vi "Simple Solenoid.vi"() -> ()   [LabVIEW 2018]
doc: "Simple Solenoid Example\n\nThis example shows how to set the value of a Solenoid Channel.\n\nIt works with the PCM (Pneumatic Control Module) communicating with the roboRIO over CAN bus. The PCM must also be supplied with 12V DC from the PDP (Power Distribution Panel).\n\nThe Compressor, Pressure Switch, and Solenoid are all wired to the PCM \n\nThis example expects a USB cable connected from your development PC to the Type B USB Jack (next to the power input) on the roboRIO.\n\nThis example expects the Driver Station to be running."
uses:
  <vilib>/Rock Robotics/WPI/Solenoid/WPI_SolenoidSetEnum.vi
  <vilib>/Rock Robotics/WPI/Solenoid/WPI_SolenoidValue.ctl
panel:
  in  "Value to Write 2":bool
  in  "stop 2":bool
  in  "Value to Write":bool
  in  "stop":bool
  # "Set this input before running."
  # "This can be set while running."
  # "On"
  # "Off"
  # "Wiring Diagram"
  # "Pneumatic Control Module"
  # "To Solenoid"
  # "CAN"
  # "COMPRESSOR OUT"
  # "PRESSURE"
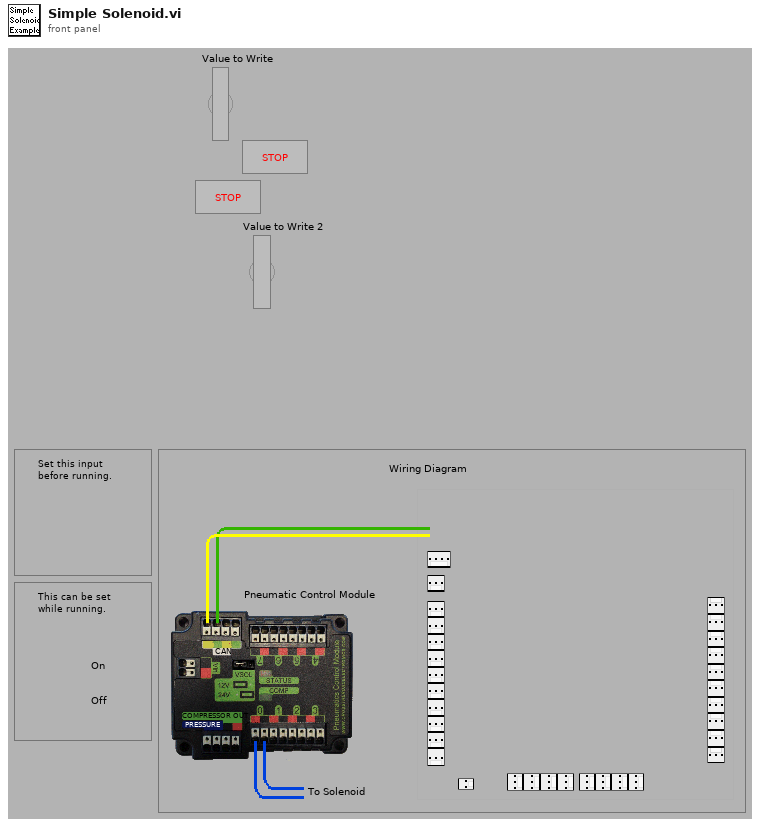
[diagram p1: front panel]
types:
  T1 = typedef "WPI_SolenoidValue.ctl" = enum16{"Off", "On", "Forward", "Reverse"}
  T2 = typedef "WPI_SolenoidDevRef.ctl" = cluster{"DevStatus":errorcluster, "Pneumatics Control Module":u8, "Forward Solenoid Channel":T3, "Reverse Solenoid Channel":T3}
  T3 = typedef "WPI_SolenoidChannel.ctl" = enum8{"Solenoid 0", "Solenoid 1", "Solenoid 2", "Solenoid 3", "Solenoid 4", "Solenoid 5", "Solenoid 6", "Solenoid 7", "Invalid"}
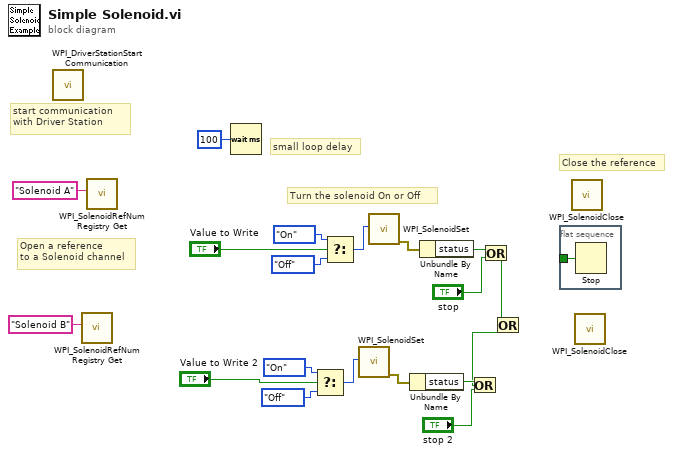
[diagram p0: block diagram]
diagram:
  # "small loop delay"
  # "Turn the solenoid On or Off"
  # "start communication with Driver Station"
  # "Close the reference"
  # "Open a reference \nto a Solenoid channel"
  n1 = call <vilib>:"WPI_DriverStationStart Communication.vi"() -> ()  [unwired: 2 in, 10 out]
  n2 = call <vilib>:"WPI_SolenoidRefNum Registry Get.vi"("refnum name"="Solenoid B") -> ("SolenoidDevRef"=w23:T2)  [unwired: 9 in, 1 out]
  n3 = call <vilib>:"WPI_SolenoidRefNum Registry Get.vi"("refnum name"="Solenoid A") -> ("SolenoidDevRef"=w26:T2)  [unwired: 9 in, 1 out]
  n4 = Wait (ms)(milliseconds to wait=u32 100) -> ()  [unwired: 1 out]
  n5 = Select(t=WPI_SolenoidValue."On" ("Value"), s="Value to Write 2", f=WPI_SolenoidValue."Off" ("Value")) -> (s? t:f=w6:T1)
  n6 = Select(t=WPI_SolenoidValue."On" ("Value"), s="Value to Write", f=WPI_SolenoidValue."Off" ("Value")) -> (s? t:f=w13:T1)
  n7 = call-poly <vilib>:"WPI_SolenoidSet.vi"("Value"=w6) -> ("error out"=w12:errorcluster, 3:"SolenoidDevRef"=w1:T2, 11:"SolenoidDevRef"=w2:T2)  [unwired: 1 in, 7 out]
  n8 = call-poly <vilib>:"WPI_SolenoidSet.vi"("Value"=w13) -> ("error out"=w19:errorcluster, 3:"SolenoidDevRef"=w20:T2, 11:"SolenoidDevRef"=w21:T2)  [unwired: 1 in, 7 out]
  n9 = Unbundle By Name(w12) -> ("status"=w11:bool)
  n10 = Unbundle By Name(w19) -> ("status"=w18:bool)
  n11 = Or(x=w11, y="stop 2") -> (x .or. y?=w5:bool)
  n12 = Or(x=w18, y="stop") -> (x .or. y?=w4:bool)
  n13 = Or(x=w4, y=w5) -> (x .or. y?=w3:bool)
  n14 = flat-sequence {
    tunnel: _ -> [w29]
    frame #0 {
      n15 = Stop(stop? (T)=w29) -> ()
    }
  }
  n16 = call <vilib>:"WPI_SolenoidClose.vi"() -> ("SolenoidDevRef"=w28:T2)  [unwired: 1 in, 10 out]
  n17 = call <vilib>:"WPI_SolenoidClose.vi"() -> ("SolenoidDevRef"=w25:T2)  [unwired: 1 in, 10 out]
